vi "ControlStyleReference.vi"() -> ()   [LabVIEW 2013]
panel:
  in  "Array 3":string[](array[string])
  out "Style ID 6":u32
  in  "Array 2":bool[](array[boolean])
  out "Style ID 5":u32
  in  "Array":dbl[](array[numeric])
  in  "String":string
  in  "Boolean":bool
  out "Style ID 4":u32
  out "Style ID 3":u32
  out "Style ID 2":u32
  out "Style ID":u32
  in  "Numeric":dbl
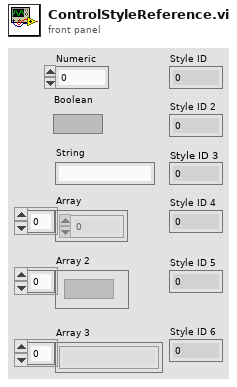
[diagram p1: front panel]
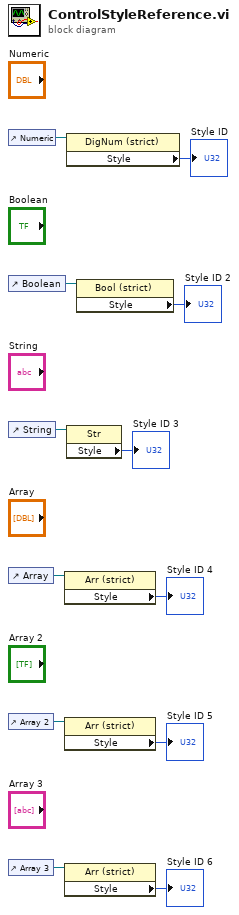
[diagram p0: block diagram]
diagram:
  n1 = control-ref of="Numeric"() -> (w12:refnum<vi>)
  n2 = control-ref of="Boolean"() -> (w7:refnum<vi>)
  n3 = control-ref of="String"() -> (w6:refnum<vi>)
  n4 = control-ref of="Array"() -> (w5:refnum<vi>)
  n5 = control-ref of="Array 2"() -> (w3:refnum<vi>)
  n6 = control-ref of="Array 3"() -> (w1:refnum<vi>)
  n7 = property class="Arr (strict)"(reference=w5) -> ("Style"=→"Style ID 4":u32)  [unwired: 1 in, 2 out]
  n8 = property class="Arr (strict)"(reference=w3) -> ("Style"=→"Style ID 5":u32)  [unwired: 1 in, 2 out]
  n9 = property class="Arr (strict)"(reference=w1) -> ("Style"=→"Style ID 6":u32)  [unwired: 1 in, 2 out]
  n10 = property class="DigNum (strict)"(reference=w12) -> ("Style"=→"Style ID":u32)  [unwired: 1 in, 2 out]
  n11 = property class="Str"(reference=w6) -> ("Style"=→"Style ID 3":u32)  [unwired: 1 in, 2 out]
  n12 = property class="Bool (strict)"(reference=w7) -> ("Style"=→"Style ID 2":u32)  [unwired: 1 in, 2 out]
